vi "verifySignatureBlobs.vi"(6 "timeout (10000)":i32=10000, 8 "error in (no error)":errorcluster, 11 "Request":T1={"random"={"method"="", "hashedApiKey"="", "n"=0, "size"=0, "format"="base64", "data"=[], "completionTime"="", "serialNumber"=0}, "signature"="", "id"=0.0}) -> (0 "error out":errorcluster, 3 "Response":T2, 4 "error data":string[](array[string]))   [LabVIEW 2014, in "Random JSON API.lvlib"]
uses:
  Random JSON API.lvlib
  Type Defs/verifySignatureResponse.ctl
  Type Defs/verifySignatureBlobsRequest.ctl
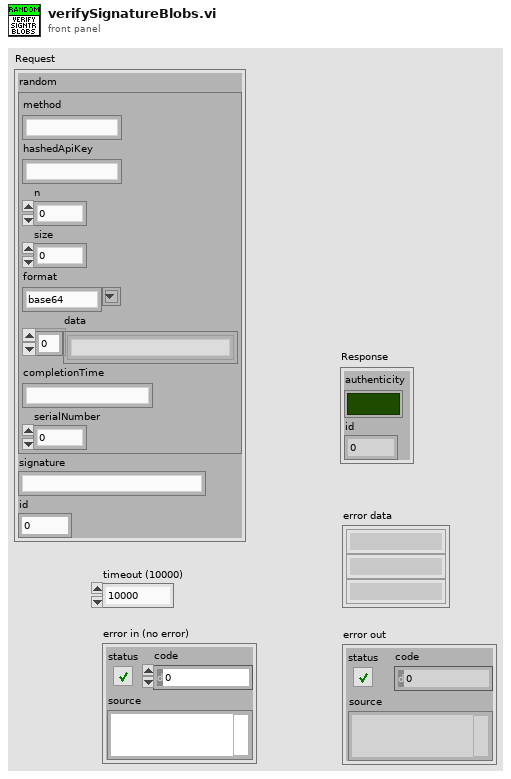
[diagram p1: front panel]
types:
  T1 = typedef "Random JSON API.lvlib/verifySignatureBlobsRequest.ctl" = cluster{"random":cluster{"method":string, "hashedApiKey":string, "n":i32, "size":i32, "format":string, "data":string[], "completionTime":string, "serialNumber":i32}, "signature":string, "id":dbl}
  T2 = typedef "Random JSON API.lvlib/verifySignatureResponse.ctl" = cluster{"authenticity":bool, "id":dbl}
  T3 = cluster{"jsonrpc":string, "method":string, "params":cluster{"random":cluster{"method":string, "hashedApiKey":string, "n":i32, "size":i32, "format":string, "data":string[], "completionTime":string, "serialNumber":i32}, "signature":string}, "id":dbl}
  T4 = cluster{"method":string, "hashedApiKey":string, "n":i32, "size":i32, "format":string, "data":string[], "completionTime":string, "serialNumber":i32}
  T5 = cluster{"random":cluster{"method":string, "hashedApiKey":string, "n":i32, "size":i32, "format":string, "data":string[], "completionTime":string, "serialNumber":i32}, "signature":string}
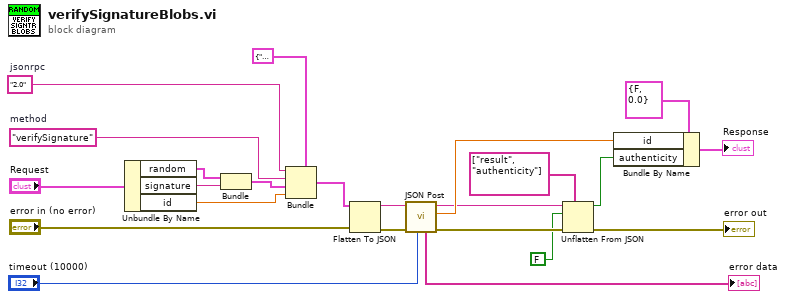
[diagram p0: block diagram]
diagram:
  w11 = "2.0"  # jsonrpc
  w10 = "verifySignature"  # method
  n1 = Unbundle By Name("Request") -> ("random"=w5:T4, "signature"=w4:string, "id"=w6:dbl)
  n2 = Bundle("random"=w5, "signature"=w4) -> (w3:T5)  [unwired: 1 in]
  n3 = Bundle(cluster=T3 {"jsonrpc"="2.0", "method"="verifySignature", "params"={"random"={"method"="", "hashedApiKey"="", "n"=0, "size"=0, "format"="base64", "data"=[], "completionTime"="", "serialNumber"=0}, "signature"=""}, "id"=0.0}, "jsonrpc"=w11, "method"=w10, "params"=w3, "id"=w6) -> (w7:T3)
  n4 = Flatten To JSON(anything=w7, error in (no error)="error in (no error)") -> (JSON string=w12:string, 11:w13:errorcluster)  [unwired: 1 in]
  n5 = call "JSON Post.vi"("timeout (10000)"="timeout (10000)", "error in (no error)"=w13, "Request JSON String"=w12) -> ("error out"=w20:errorcluster, "id"=w21:dbl, "Response JSON String"=w16:string, "error data"=→"error data":string[])  [unwired: 5 in]
  n6 = Unflatten From JSON(path=string[] ["result", "authenticity"], JSON string=w16, type and defaults=FALSE, error in (no error)=w20) -> (value=w18:bool, error out=→"error out":errorcluster)  [unwired: 3 in]
  n7 = Bundle By Name(cluster=T2 {"authenticity"=FALSE, "id"=0.0} ("Response"), "id"=w21, "authenticity"=w18) -> (→"Response":T2)
